vi "Goto.vi"(6 "Home?":bool, 7 "Speed":i32, 8 "error in (no error)":errorcluster, 9 "channel":i32(ring)=1 items=["Channel1"=1, "Channel2"=2, "Channel3"=3, "Channel4"=4], 10 "New Position":sgl, 11 "Jiaxin_Stepper_Controller.lvlib:Jiaxin_Stepper.lvclass":refnum<class "Jiaxin_Stepper.lvclass">) -> (0 "error out":errorcluster, 3 "Jiaxin_Stepper_Controller.lvlib:Jiaxin_Stepper.lvclass":refnum<class "Jiaxin_Stepper.lvclass">)   [LabVIEW 2023, in "Jiaxin_Stepper_Controller.lvlib" / "Jiaxin_Stepper.lvclass"]
uses:
  Jiaxin_Stepper/Jiaxin_Stepper.lvclass
  C:/Program Files/National Instruments/LabVIEW 2023/vi.lib/ActorFramework/Actor/Actor.lvclass
  UIs/TranslationStage_UI/TranslationStage_UI/StageMoveDone_For_UI.ctl
  Jiaxin_Stepper/Jiaxin_Stepper.lvclass/Jiaxin_Stepper.ctl
  <vilib>/ActorFramework/Actor/Actor.lvclass/Actor.ctl
  Interfaces/AbstractInstrumentClasses/TranslationStages_LV/TranslationStagesComm Messages/StageMoveDone Msg/StageMoveDone Msg.lvclass/StageMoveDone Msg.ctl
  <vilib>/ActorFramework/Message Enqueuer/Message Enqueuer.lvclass/Message Enqueuer.ctl
  <vilib>/ActorFramework/Message Enqueuer/Enqueue.vi
  Interfaces/AbstractInstrumentClasses/TranslationStages_LV/TranslationStagesComm Messages/StageMoveDone Msg/StageMoveDone Msg.lvclass
  C:/Program Files/National Instruments/LabVIEW 2023/vi.lib/ActorFramework/Message/Message.lvclass
  <vilib>/ActorFramework/Message Priority Queue/Priority Enqueue.vi
  Jiaxin_Stepper_Controller.lvlib
  <vilib>/ActorFramework/Actor/Actor.lvclass
  typedefs/typedefs.lvlib
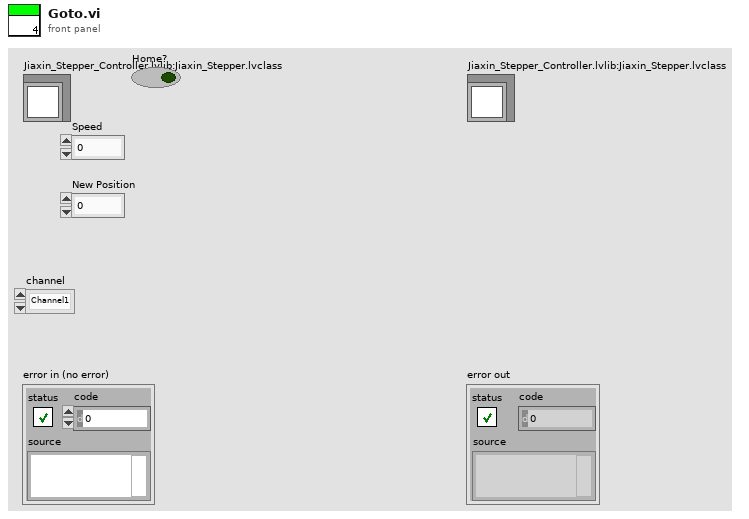
[diagram p1: front panel]
types:
  T1 = typedef "typedefs.lvlib/StageMoveDone_For_UI.ctl" = cluster{"CH1 Pos":sgl, "CH2 Pos":dbl, "CH3 Pos":dbl, "CH4 Pos":dbl, "Home?":bool}
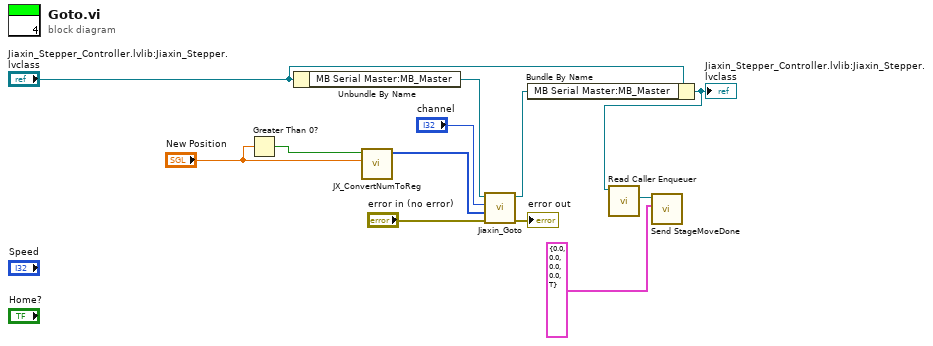
[diagram p0: block diagram]
diagram:
  n1 = Greater Than 0?(x="New Position") -> (x > 0?=w8:bool)
  n2 = Unbundle By Name("Jiaxin_Stepper_Controller.lvlib:Jiaxin_Stepper.lvclass") -> ("MB Serial Master:MB_Master"=w5:refnum<class "MB_Master.lvclass">)
  n3 = call "JX_ConvertNumToReg.vi"("Steps"="New Position", "Direction"=w8) -> ("Array"=w10:u16[])  [unwired: 9 in]
  n4 = call "Jiaxin_Goto.vi"("error in (no error)"="error in (no error)", "Abs Position Registers"=w10, "Channel"="channel", "MB Serial Master:MB_Master"=w5) -> ("error out"=→"error out":errorcluster, "MB Serial Master:MB_Master"=w6:refnum<class "MB_Master.lvclass">)  [unwired: 6 in]
  n5 = Bundle By Name(cluster="Jiaxin_Stepper_Controller.lvlib:Jiaxin_Stepper.lvclass", "MB Serial Master:MB_Master"=w6) -> (w1:refnum<class "Jiaxin_Stepper.lvclass">)
  "Jiaxin_Stepper_Controller.lvlib:Jiaxin_Stepper.lvclass" <- w1
  n6 = call <vilib>:"Read Caller Enqueuer.vi"("Actor"=w1) -> ("Caller Enqueuer"=w3:refnum<class "Message Enqueuer.lvclass">)  [unwired: 10 in]
  n7 = call "Send StageMoveDone.vi"("Positions"=T1 {"CH1 Pos"=0.0, "CH2 Pos"=0.0, "CH3 Pos"=0.0, "CH4 Pos"=0.0, "Home?"=TRUE}, "Message Enqueuer"=w3) -> ()  [unwired: 8 in, 2 out]
